vi "Test Load Instruments 2.vi"(11 "Test Case In":refnum<class "Test Instrument Manager.lvclass">) -> (0 "error out":errorcluster, 3 "Test Case Out":refnum<class "Test Instrument Manager.lvclass">)   [LabVIEW 2025, in "Test Instrument Manager.lvclass"]
uses:
  Test Instrument Manager.lvclass
  <vilib>/Astemes/LUnit/Test Case.lvclass/Test Case.ctl
  <vilib>/Astemes/LUnit/Core/LUnit Test Case/Private/Append Pass Result.vi
  <vilib>/Astemes/LUnit/Core/LUnit Test Case/Private/Append Fail Result.vi
  <vilib>/Astemes/LUnit/Core/LUnit Test Case/Private/Run In UI.vi
  <vilib>/Utility/error.llb/Clear Errors.vi
  Instrument Manager/Instrument Manager.lvclass
  <vilib>/Astemes/LUnit/Test Case.lvclass
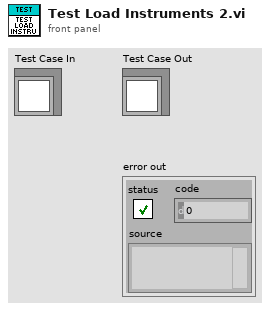
[diagram p1: front panel]
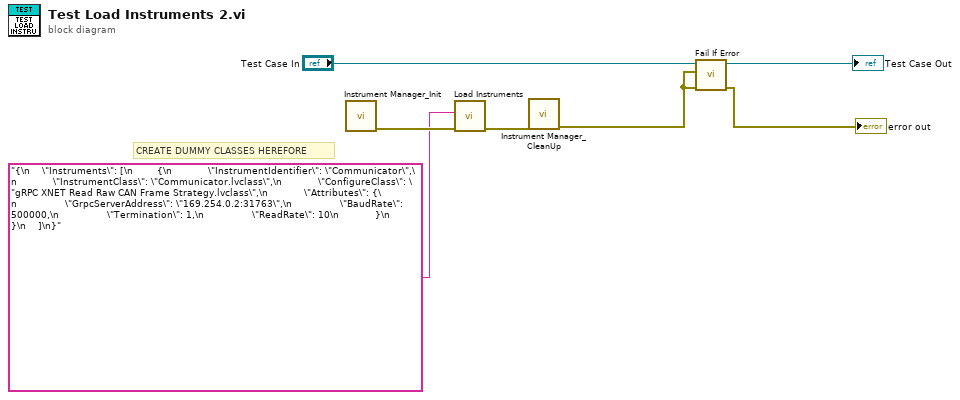
[diagram p0: block diagram]
diagram:
  # "CREATE DUMMY CLASSES HEREFORE"
  n1 = call "Instrument Manager_Init.vi"() -> ("Error Out"=w5:errorcluster)  [unwired: 10 in, 1 out]
  n2 = call "Load Instruments.vi"("Error In"=w5, "Source"="{\n    \"Instruments\": [\n        {\n            \"InstrumentIdentifier\": \"Communicator\",\n            \"InstrumentClass\": \"Communicator.lvclass\",\n            \"ConfigureClass\": \"gRPC XNET Read Raw CAN Frame Strategy.lvclass\",\n            \"Attributes\": {\n                \"GrpcServerAddress\": \"169.254.0.2:31763\",\n                \"BaudRate\": 500000,\n                \"Termination\": 1,\n                \"ReadRate\": 10\n            }\n        }\n    ]\n}") -> ("Error Out"=w4:errorcluster)  [unwired: 9 in]
  n3 = call "Instrument Manager_CleanUp.vi"("Error In"=w4) -> ("Error Out"=w1:errorcluster)  [unwired: 10 in]
  n4 = call <vilib>:"Fail If Error.vi"("error in (no error)"=w1, "Assert error"=w1, "LUnit Test Case In"="Test Case In") -> ("error out"=→"error out":errorcluster, "LUnit Test Case Out"=→"Test Case Out":refnum<class "Test Instrument Manager.lvclass">)  [unwired: 7 in]
